vi "SIMDMM_Timestamp Subtract.vi"(1 "y":timestamp format="%<%X\n%x>T", 2 "x":timestamp format="%<%X\n%x>T") -> (0 "x - y":timestamp format="%<%X\n%x>T")   [LabVIEW 2019]
uses:
  SIMDMM_I128 Timestamp.ctl
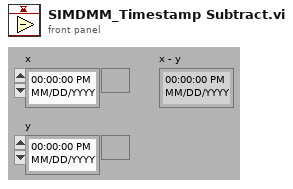
[diagram p1: front panel]
types:
  T1 = typedef "SIMDMM_I128 Timestamp.ctl" = cluster{"high":i32, "mid high":u32, "mid low":u32, "low":u32}
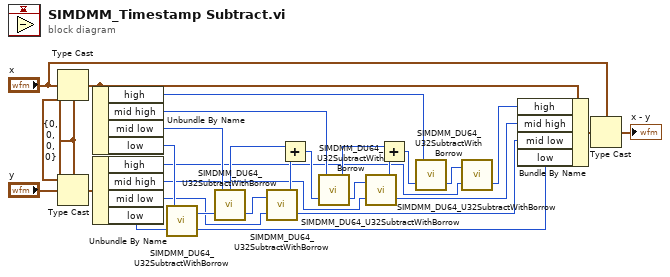
[diagram p0: block diagram]
diagram:
  w1 = T1 {"high"=0, "mid high"=0, "mid low"=0, "low"=0} ("timestamp")
  n1 = Type Cast(type=w1, x="x") -> (*(type *) &x=w3:T1)
  n2 = Type Cast(type=w1, x="y") -> (*(type *) &x=w2:T1)
  n3 = Unbundle By Name(w3) -> ("high"=w7:i32, "mid high"=w9:u32, "mid low"=w14:u32, "low"=w27:u32)
  n4 = Unbundle By Name(w2) -> ("high"=w8:i32, "mid high"=w11:u32, "mid low"=w12:u32, "low"=w28:u32)
  n5 = call "SIMDMM_DU64_U32SubtractWithBorrow.vi"("y"=w28, "x"=w27) -> ("x - y"=w26:u32, "borrow"=w25:u32)
  n6 = call "SIMDMM_DU64_U32SubtractWithBorrow.vi"("y"=w25, "x"=w14) -> ("x - y"=w13:u32, "borrow"=w22:u32)
  n7 = call "SIMDMM_DU64_U32SubtractWithBorrow.vi"("y"=w12, "x"=w13) -> ("x - y"=w24:u32, "borrow"=w23:u32)
  n8 = Add(x=w22, y=w23) -> (x+y=w21:u32)
  n9 = call "SIMDMM_DU64_U32SubtractWithBorrow.vi"("y"=w21, "x"=w9) -> ("x - y"=w10:u32, "borrow"=w18:u32)
  n10 = call "SIMDMM_DU64_U32SubtractWithBorrow.vi"("y"=w11, "x"=w10) -> ("x - y"=w20:u32, "borrow"=w19:u32)
  n11 = Add(x=w18, y=w19) -> (x+y=w17:u32)
  n12 = call "SIMDMM_DU64_U32SubtractWithBorrow.vi"("y"=w17, "x"=w7) -> ("x - y"=w6:u32)  [unwired: 1 out]
  n13 = call "SIMDMM_DU64_U32SubtractWithBorrow.vi"("y"=w8, "x"=w6) -> ("x - y"=w16:u32)  [unwired: 1 out]
  n14 = Bundle By Name(cluster=w3, "high"=w16, "mid high"=w20, "mid low"=w24, "low"=w26) -> (w15:T1)
  n15 = Type Cast(type="x", x=w15) -> (*(type *) &x=→"x - y":timestamp)
